vi "WILT Format Summary File.vi"(11 "WILT Summary Cluster Input":T1) -> (3 "Summary Data":string[](array[string]))   [LabVIEW 2016]
uses:
  Type Definitions/WILT Summary Data.ctl
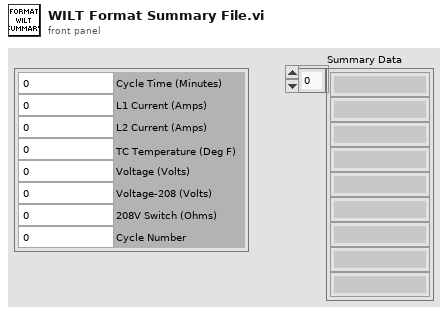
[diagram p1: front panel]
types:
  T1 = typedef "WILT Summary Data.ctl" = cluster{"Cycle Time (Minutes)":dbl, "L1 Current (Amps)":dbl, "L2 Current (Amps)":dbl, "TC Temperature (Deg F)":dbl, "Voltage (Volts)":dbl, "Voltage-208 (Volts)":dbl, "208V Switch (Ohms)":dbl, "Cycle Number":i32}
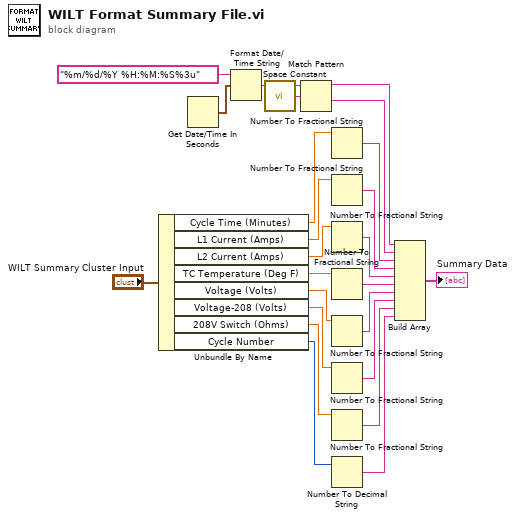
[diagram p0: block diagram]
diagram:
  n1 = Unbundle By Name("WILT Summary Cluster Input") -> ("Cycle Time (Minutes)"=w19:dbl, "L1 Current (Amps)"=w18:dbl, "L2 Current (Amps)"=w17:dbl, "TC Temperature (Deg F)"=w16:dbl, "Voltage (Volts)"=w15:dbl, "Voltage-208 (Volts)"=w14:dbl, "208V Switch (Ohms)"=w13:dbl, "Cycle Number"=w2:i32)
  n2 = Get Date/Time In Seconds() -> (seconds since 1Jan1904=w21:timestamp)
  n3 = Format Date/Time String(time format string (%c)="%m/%d/%Y %H:%M:%S%3u", seconds (now)=w21) -> (date/time string=w23:string)  [unwired: 1 in]
  n4 = call <vilib>:"Space Constant.vi"() -> ("String"=w24:string)
  n5 = Match Pattern(string=w23, regular expression=w24) -> (before substring=w12:string, after substring=w11:string)  [unwired: 1 in, 2 out]
  n6 = Number To Fractional String(number=w19) -> (F-format string=w10:string)  [unwired: 3 in]
  n7 = Number To Fractional String(number=w18) -> (F-format string=w9:string)  [unwired: 3 in]
  n8 = Number To Fractional String(number=w17) -> (F-format string=w8:string)  [unwired: 3 in]
  n9 = Number To Fractional String(number=w16) -> (F-format string=w7:string)  [unwired: 3 in]
  n10 = Number To Fractional String(number=w15) -> (F-format string=w6:string)  [unwired: 3 in]
  n11 = Number To Fractional String(number=w14) -> (F-format string=w5:string)  [unwired: 3 in]
  n12 = Number To Fractional String(number=w13) -> (F-format string=w4:string)  [unwired: 3 in]
  n13 = Number To Decimal String(number=w2) -> (decimal integer string=w1:string)  [unwired: 1 in]
  n14 = Build Array(w12, w11, w10, w9, w8, w7, w6, w5, w4, w1) -> (→"Summary Data":string[])
